vi "Parameter Type to String.vi"(0 "String in":string, 5 "Message Name":string, 7 "Parameters":T1[](array[typedef])) -> (4 "String out":string)   [LabVIEW 2011, in "AIT 1553 Custom Device.lvlib"]
uses:
  Controls/1553 Param.ctl
  AIT 1553 Custom Device.lvlib
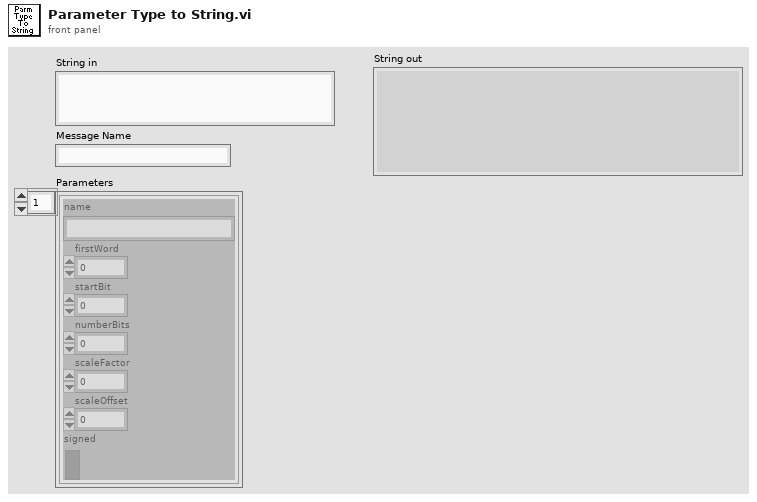
[diagram p1: front panel]
types:
  T1 = typedef "AIT 1553 Custom Device.lvlib/1553 Param.ctl" = cluster{"name":string, "firstWord":i32, "startBit":i32, "numberBits":i32, "scaleFactor":dbl, "scaleOffset":dbl, "signed":bool}
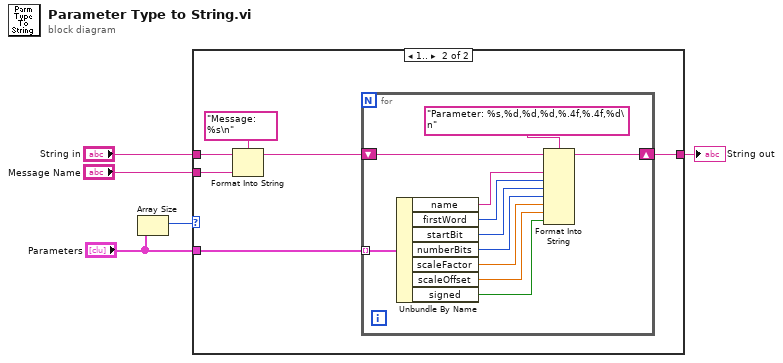
[diagram p0: block diagram]
diagram:
  n1 = Array Size(array="Parameters") -> (size(s)=w1:i32)
  n2 = case shown="1.." w1 {
    tunnel: [w6 w12] -> w5
    tunnel: "String in" -> [w6 w9]
    tunnel: "Parameters" -> [_ w11]
    tunnel: "Message Name" -> [_ w7]
    frame Default {
    }
    frame 1.. {
      n3 = Format Into String(format string="Message: %s\n", initial string=w9, w7) -> (resulting string=w8:string)  [unwired: 1 in, 1 out]
      n4 = for {
        tunnel: w11 -> [w23] mode=indexing
        shift-right: [w20] -> w12
        shift-left: w8 -> [w21]
        n5 = Unbundle By Name(w23) -> ("name"=w19:string, "firstWord"=w18:i32, "startBit"=w17:i32, "numberBits"=w16:i32, "scaleFactor"=w15:dbl, "scaleOffset"=w14:dbl, "signed"=w13:bool)
        n6 = Format Into String(format string="Parameter: %s,%d,%d,%d,%.4f,%.4f,%d\n", initial string=w21, w19, w18, w17, w16, w15, w14, w13) -> (resulting string=w20:string)  [unwired: 1 in, 1 out]
      }
    }
  }
  "String out" <- w5
